vi "RANGE Gas Lab Flow Calc.vi"(0 "Meter Data":T1={"Meter Size"=0.0, "DAQ Output (Voltage)"=0.0, "Reference (Voltage)"=0.0, "Meter Present"=FALSE, "Meter Visa"="COM3", "Gas Type"="", "SLPM Error @ Zero"=0.0, "Gas Mix Number"="", "Set STP Register"=FALSE, "Measurement Units"={"Abs. Pressure"="", "Gauge/Diff. Press."="", "Barometric Press."="", "Temperature"="", "Volume"="", "Mass"="", "Setpoint"="", "Valve Drive"="", "Totalizer"="", "Tot. Timer"="", "Tot. Avg. Flow"="", "Tot. Peak Flow"="", "Software Version"=""}}, 5 "Error In":errorcluster, 7 "Heating Value (BTU/ft³)":dbl) -> (14 "Ft³/Hr (SCFH)":dbl, 15 "BTU/Hr":dbl, 18 "SLPM":dbl, 19 "Error Out":errorcluster)   [LabVIEW 2016]
uses:
  Type Definitions/RANGE DAQ Data.ctl
  Drivers/Omega FMA-1600A Series Gas Flow Meter/Type Definitions/FMA1600A Gas Type.ctl
  Drivers/Omega FMA-1600A Series Gas Flow Meter/Type Definitions/FMA1600A Units String.ctl
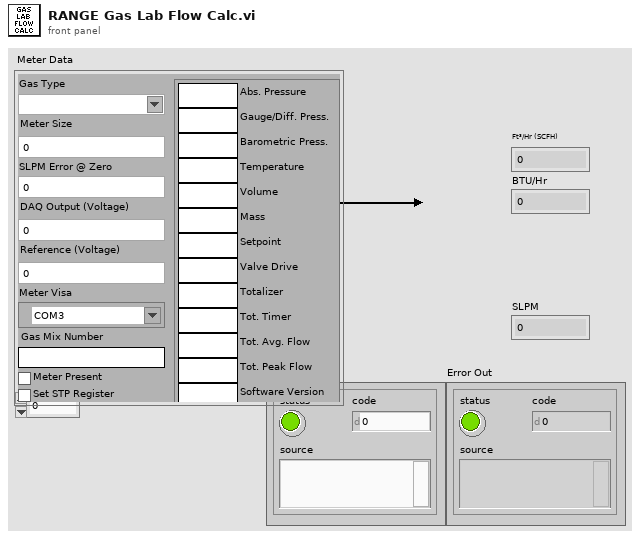
[diagram p1: front panel]
types:
  T1 = typedef "RANGE DAQ Data.ctl" = cluster{"Meter Size":dbl, "DAQ Output (Voltage)":dbl, "Reference (Voltage)":dbl, "Meter Present":bool, "Meter Visa":refnum<visa-resource-name>, "Gas Type":T2, "SLPM Error @ Zero":dbl, "Gas Mix Number":string, "Set STP Register":bool, "Measurement Units":T3}
  T2 = typedef "FMA1600A Gas Type.ctl" = string
  T3 = typedef "FMA1600A Units String.ctl" = cluster{"Abs. Pressure":string, "Gauge/Diff. Press.":string, "Barometric Press.":string, "Temperature":string, "Volume":string, "Mass":string, "Setpoint":string, "Valve Drive":string, "Totalizer":string, "Tot. Timer":string, "Tot. Avg. Flow":string, "Tot. Peak Flow":string, "Software Version":string}
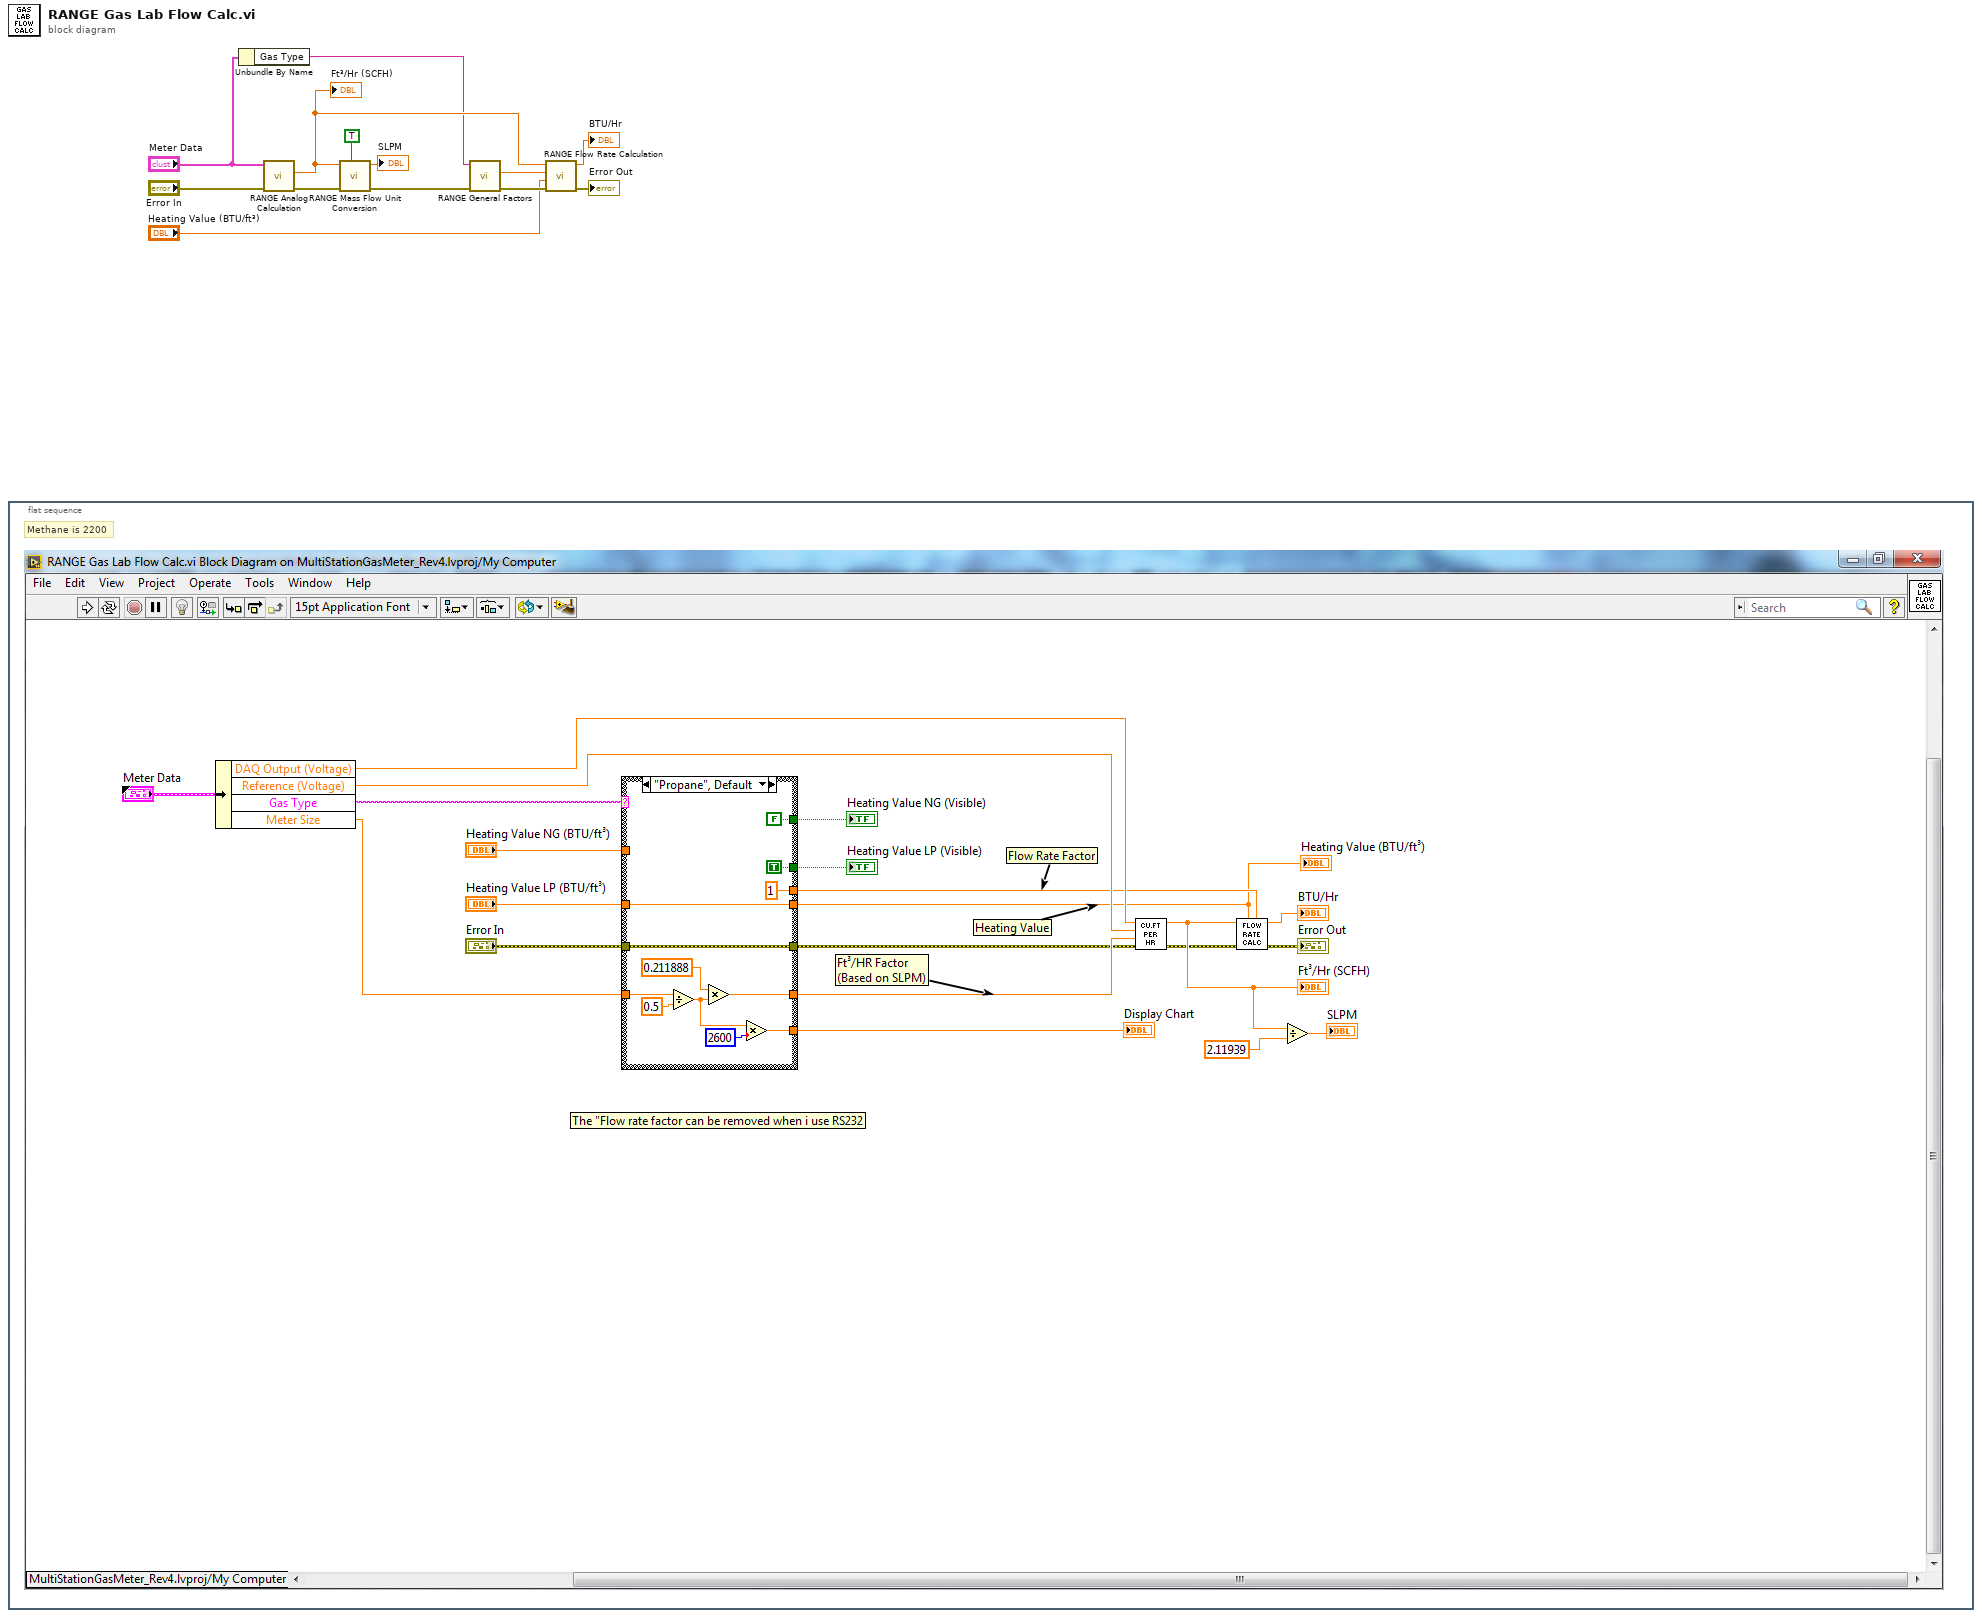
[diagram p0: block diagram]
diagram:
  n1 = flat-sequence {
    frame #0 {
      # "Methane is 2200"
    }
  }
  n2 = Unbundle By Name("Meter Data") -> ("Gas Type"=w2:T2)
  n3 = call "RANGE Analog Calculation.vi"("error in (no error)"="Error In", "Meter Data"="Meter Data") -> ("error out"=w6:errorcluster, "Ft³/HR"=w5:dbl)  [unwired: 8 in]
  "Ft³/Hr (SCFH)" <- w5
  n4 = call "RANGE Mass Flow Unit Conversion.vi"("Ft³/HR -SLPM (T)"=TRUE, "Error In"=w6, "Input Mass Flow Rate"=w5) -> ("Error Out"=w4:errorcluster, "Output Mass Flow Rate"=→"SLPM":dbl)  [unwired: 7 in]
  n5 = call "RANGE General Factors.vi"("Error In"=w4, "Gas Type String"=w2) -> ("Error Out"=w10:errorcluster, "Flow Rate Factor"=w9:dbl)  [unwired: 8 in]
  n6 = call "RANGE Flow Rate Calculation.vi"("Error In"=w10, "Heating Value (BTU/ft³)"="Heating Value (BTU/ft³)", "Flow Rate Factor"=w9, "Ft³/HR"=w5) -> ("Error Out"=→"Error Out":errorcluster, "Flow Rate (BTU/Hr)"=→"BTU/Hr":dbl)  [unwired: 6 in]
